vi "DashboardGetVariable.vi"(8 "Dashboard":refnum<k24>, 9 "name":string, 11 "error in":errorcluster) -> (0 "Response":cluster{"Message":string, "Succeed":bool}, 1 "Value":T1, 3 "error out":errorcluster)   [LabVIEW 2023, in "UnderAutomation.UniversalRobots.lvlib"]
uses:
  UnderAutomation.UniversalRobots.lvlib
  C:/Users/fg/Documents/UniversalRobots.vi/UnderAutomation.UniversalRobots/lib/UnderAutomation.UniversalRobots.dll
  lib/UnderAutomation.UniversalRobots.dll
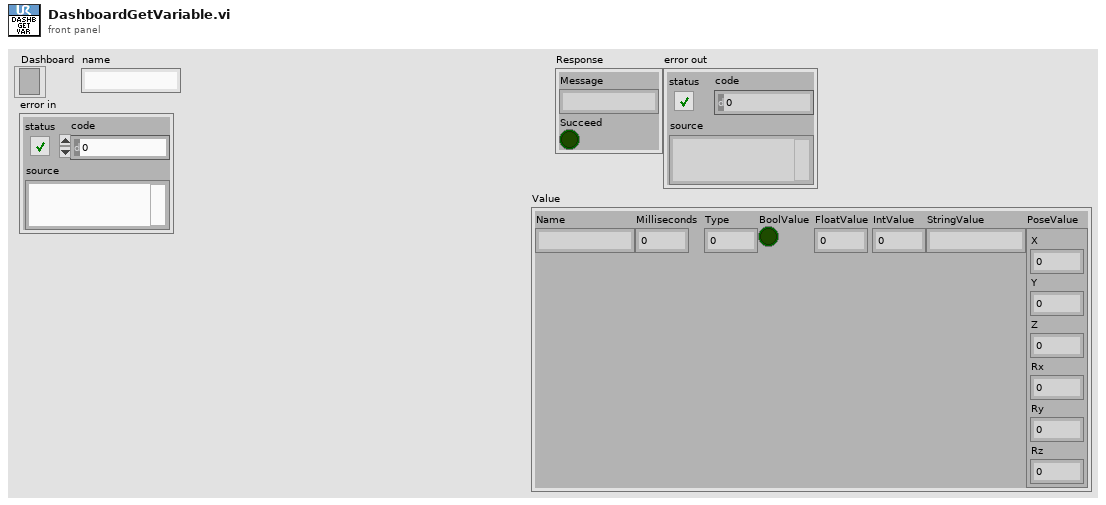
[diagram p1: front panel]
types:
  T1 = cluster{"Name":string, "Milliseconds":i32, "Type":i32, "BoolValue":bool, "FloatValue":sgl, "IntValue":i32, "StringValue":string, "PoseValue":cluster{"X":dbl, "Y":dbl, "Z":dbl, "Rx":dbl, "Ry":dbl, "Rz":dbl}}
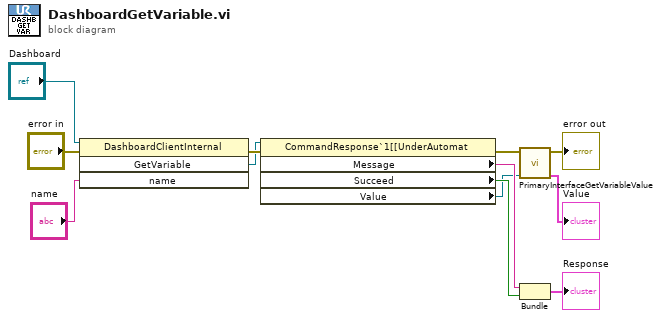
[diagram p0: block diagram]
diagram:
  n1 = invoke class="DashboardClientInternal" method="GetVariable"(reference="Dashboard", error in="error in", "name"="name") -> (error out=w7:errorcluster, "GetVariable"=w1:refnum<k24>)  [unwired: 1 in, 2 out]
  n2 = property class="CommandResponse`1[[UnderAutomat"(reference=w1, error in=w7) -> (error out=w4:errorcluster, "Message"=w11:string, "Succeed"=w10:bool, "Value"=w5:refnum<k24>)  [unwired: 1 out]
  n3 = call "PrimaryInterfaceGetVariableValue.vi"("Variable"=w5, "error in"=w4) -> ("Value"=→"Value":T1, "error out"=→"error out":errorcluster)  [unwired: 8 in]
  n4 = Bundle("Message"=w11, "Succeed"=w10) -> (→"Response":cluster{"Message":string, "Succeed":bool})  [unwired: 1 in]
